vi "Get Combo Value.vi"(7 "Register Map":T1, 11 "Operand":i32) -> (3 "Combo Value":i32)   [LabVIEW 2024]
uses:
  MAP_Registers.ctl
  ENUM_Combo Select.ctl
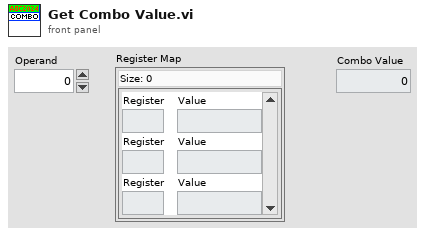
[diagram p1: front panel]
types:
  T1 = typedef "MAP_Registers.ctl" = map{string, i32}
  T2 = typedef "ENUM_Combo Select.ctl" = enum16{"0", "1", "2", "3", "A", "B", "C", "XXX"}
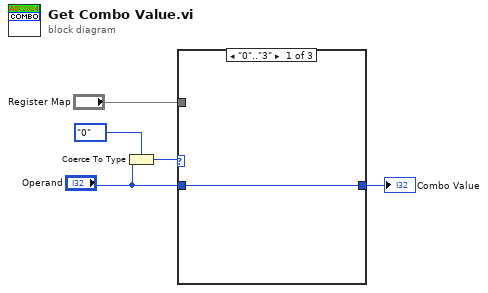
[diagram p0: block diagram]
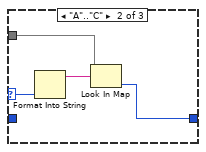
[diagram p2: hidden frame]
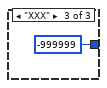
[diagram p3: hidden frame]
diagram:
  n1 = Coerce To Type(0:"Operand", 1:ENUM_Combo_Select."0" ("Combo Values")) -> (2:w4:T2)
  n2 = case shown="\"0\"..\"3\"" w4 {
    selector: w4 -> [_ w9 _]
    tunnel: "Operand" -> [w6 _ _]
    tunnel: [w6 w7 -999999 ("Operand")] -> w2
    tunnel: "Register Map" -> [_ w10 _]
    frame "0".."3" {
    }
    frame "A".."C" {
      n3 = Format Into String(w9) -> (resulting string=w8:string)  [unwired: 3 in, 1 out]
      n4 = Look In Map(map=w10, key=w8) -> (value=w7:i32)  [unwired: 1 in, 1 out]
    }
    frame "XXX" {
    }
  }
  "Combo Value" <- w2
